vi "Conversion_Simple.vi"(5 "Input = DBL/String (DBL[false])":bool, 6 "Microsteps (MS=64)":dbl=64.0, 7 "Motor":u16(ring)=3 items=["none", "1", "2", "3", "4", "all"], 8 "Output Unit":T1=enum."Angle [TMC]", 9 "Input Unit":T1=enum."Inches", 10 "Input String":string="0", 11 "Input":dbl format="%#_13g") -> (2 "Output":string="0", 3 "Output":dbl)   [LabVIEW 2018]
uses:
  ConversionAndInformation/Unit_Control.ctl
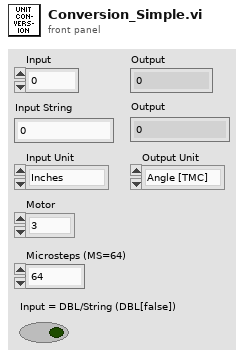
[diagram p1: front panel]
types:
  T1 = typedef "Unit_Control.ctl" = enum16{"Angle (Degrees)", "Rad", "Angle [TMC]", "Microsteps [TMC]", "Inches", "Nanometer", "Meter", "Centimeter", "Millimeter", "Micron"}
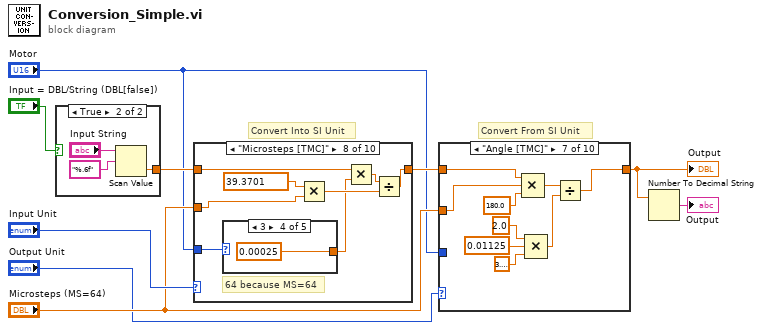
[diagram p0: block diagram]
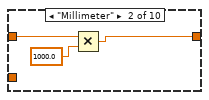
[diagram p3: hidden frame]
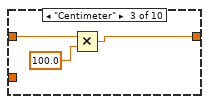
[diagram p4: hidden frame]
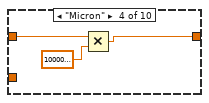
[diagram p5: hidden frame]
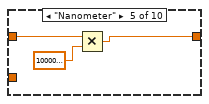
[diagram p6: hidden frame]
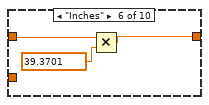
[diagram p7: hidden frame]
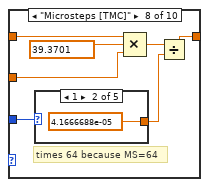
[diagram p8: hidden frame]
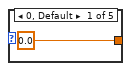
[diagram p9: hidden frame]
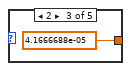
[diagram p10: hidden frame]
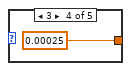
[diagram p11: hidden frame]
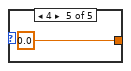
[diagram p12: hidden frame]
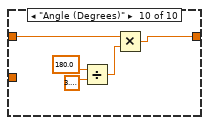
[diagram p14: hidden frame]
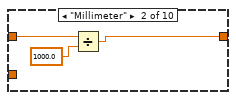
[diagram p16: hidden frame]
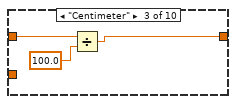
[diagram p17: hidden frame]
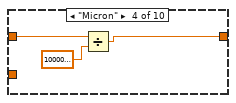
[diagram p18: hidden frame]
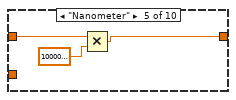
[diagram p19: hidden frame]
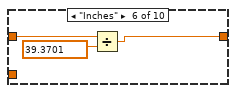
[diagram p20: hidden frame]
diagram:
  # "Convert From SI Unit"
  # "Convert Into SI Unit"
  n1 = case shown="True" "Input = DBL/String (DBL[false])" {
    tunnel: ["Input" w11] -> w6
    frame False {
    }
    frame True {
      n2 = Scan Value(string="Input String", format string="%.6f") -> (value=w11:dbl)  [unwired: 1 in, 1 out]
    }
  }
  n3 = case shown="\"Microsteps [TMC]\"" "Input Unit" {
    tunnel: w6 -> [w14 w17 w20 w23 w26 w28 w38 w44 w53 w56]
    tunnel: [w14 w16 w18 w22 w24 w27 w37 w43 w53 w54] -> w5
    tunnel: "Motor" -> [_ _ _ _ _ _ _ w42 _ _]
    tunnel: "Microsteps (MS=64)" -> [_ _ _ _ _ _ w30 w41 _ _]
    frame "Meter", Default {
    }
    frame "Millimeter" {
      n4 = Divide(x=w17, y=1000.0) -> (x/y=w16:dbl)
    }
    frame "Centimeter" {
      n5 = Divide(x=w20, y=100.0) -> (x/y=w18:dbl)
    }
    frame "Micron" {
      n6 = Divide(x=w23, y=1000000.0) -> (x/y=w22:dbl)
    }
    frame "Nanometer" {
      n7 = Multiply(x=w26, y=1000000000.0) -> (x*y=w24:dbl)
    }
    frame "Inches" {
      n8 = Divide(x=w28, y=39.3701) -> (x/y=w27:dbl)
    }
    frame "Angle [TMC]" {
      # "only for\nmotor 4"
      # "64 because MS=64"
      n9 = Divide(x=3.141592653589793, y=180.0) -> (x/y=w32:dbl)
      n10 = Compound Arithmetic op=MULTIPLY(2.0 ("x"), 0.01125, w32) -> (w31:dbl)
      n11 = Multiply(x=w38, y=w31) -> (x*y=w39:dbl)
      n12 = Divide(x=w39, y=w30) -> (x/y=w37:dbl)
    }
    frame "Microsteps [TMC]" {
      # "64 because MS=64"
      n13 = case shown="3" w42 {
        tunnel: [0.0 4.1666688e-05 4.1666688e-05 0.00025 0.0225] -> w40
        frame 0, Default {
        }
        frame 1 {
        }
        frame 2 {
        }
        frame 3 {
        }
        frame 4 {
        }
      }
      n14 = Multiply(x=39.3701, y=w41) -> (x*y=w45:dbl)
      n15 = Multiply(x=w44, y=w40) -> (x*y=w47:dbl)
      n16 = Divide(x=w47, y=w45) -> (x/y=w43:dbl)
    }
    frame "Rad" {
    }
    frame "Angle (Degrees)" {
      n17 = Divide(x=3.141592653589793, y=180.0) -> (x/y=w55:dbl)
      n18 = Multiply(x=w56, y=w55) -> (x*y=w54:dbl)
    }
  }
  n19 = case shown="\"Angle [TMC]\"" "Output Unit" {
    tunnel: w5 -> [w59 w62 w65 w68 w71 w73 w83 w88 w96 w99]
    tunnel: [w59 w61 w63 w67 w70 w72 w79 w87 w96 w97] -> w1
    tunnel: "Motor" -> [_ _ _ _ _ _ _ w86 _ _]
    tunnel: "Microsteps (MS=64)" -> [_ _ _ _ _ _ w75 w85 _ _]
    frame "Meter", Default {
    }
    frame "Millimeter" {
      n20 = Multiply(x=w62, y=1000.0) -> (x*y=w61:dbl)
    }
    frame "Centimeter" {
      n21 = Multiply(x=w65, y=100.0) -> (x*y=w63:dbl)
    }
    frame "Micron" {
      n22 = Multiply(x=w68, y=1000000.0) -> (x*y=w67:dbl)
    }
    frame "Nanometer" {
      n23 = Multiply(x=w71, y=1000000000.0) -> (x*y=w70:dbl)
    }
    frame "Inches" {
      n24 = Multiply(x=w73, y=39.3701) -> (x*y=w72:dbl)
    }
    frame "Angle [TMC]" {
      n25 = Compound Arithmetic op=MULTIPLY(w83, w75, 180.0 ("y")) -> (w81:dbl)
      n26 = Compound Arithmetic op=MULTIPLY(2.0 ("x"), 0.01125, 3.141592653589793) -> (w80:dbl)
      n27 = Divide(x=w81, y=w80) -> (x/y=w79:dbl)
    }
    frame "Microsteps [TMC]" {
      # "times 64 because MS=64"
      n28 = case shown="1" w86 {
        tunnel: [0.0 4.1666688e-05 4.1666688e-05 0.00025 0.0] -> w84
        frame 0, Default {
        }
        frame 1 {
        }
        frame 2 {
        }
        frame 3 {
        }
        frame 4 {
        }
      }
      n29 = Compound Arithmetic op=MULTIPLY(w88, 39.3701, w85) -> (w89:dbl)
      n30 = Divide(x=w89, y=w84) -> (x/y=w87:dbl)
    }
    frame "Rad" {
    }
    frame "Angle (Degrees)" {
      n31 = Divide(x=180.0 ("y"), y=3.141592653589793) -> (x/y=w98:dbl)
      n32 = Multiply(x=w99, y=w98) -> (x*y=w97:dbl)
    }
  }
  "Output" <- w1
  n33 = Number To Decimal String(number=w1) -> (decimal integer string=→"Output":string)  [unwired: 1 in]
